vi "Position String to right of previous.vi"(6 "Units":refnum<vi>, 8 "error in (no error)":errorcluster, 10 "Prev String Ref":refnum<vi>, 11 "String Ref":refnum<vi>) -> (0 "Error Out":errorcluster)   [LabVIEW 2014]
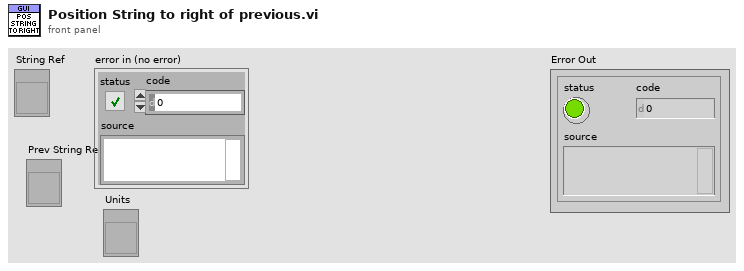
[diagram p1: front panel]
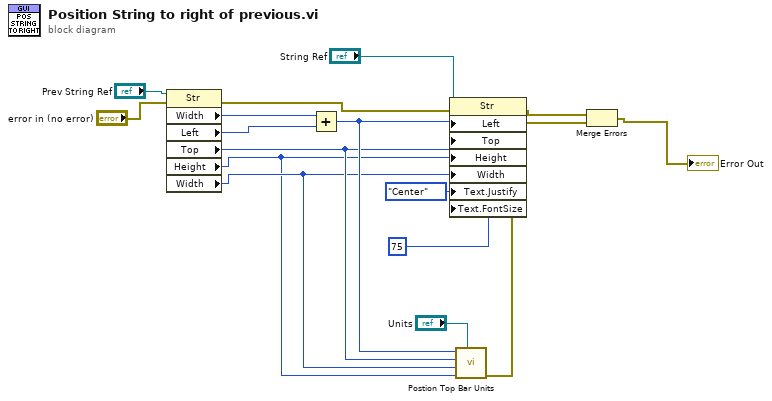
[diagram p0: block diagram]
diagram:
  n1 = property class="Str"(reference="Prev String Ref", error in="error in (no error)") -> (error out=w11:errorcluster, "Width"=w13:u32, "Left"=w14:i32, "Top"=w6:i32, "Height"=w4:u32, "Width"=w5:u32)  [unwired: 1 out]
  n2 = Add(x=w13, y=w14) -> (x+y=w7:u32)
  n3 = property class="Str"(reference="String Ref", error in=w11, "Left"=w7, "Top"=w6, "Height"=w4, "Width"=w5, "Text.Justify"=enum16{"Left", "Center", "Right"}."Center" ("Text.Justification"), "Text.FontSize"=u32 75 ("Text.Font:Size")) -> (error out=w3:errorcluster)  [unwired: 1 out]
  n4 = call "Postion Top Bar Units.vi"("Units"="Units", "Button Size:Height"=w4, "Button Witdh"=w5, "Top (numeric indicator)"=w6, "Left (numeric indicator)"=w7) -> ("error out"=w2:errorcluster)  [unwired: 6 in]
  n5 = Merge Errors(w3, w2) -> (→"Error Out":errorcluster)
